vi "ma_Tone estimation (FFT input).vi"(1 "spectral info":T1 {"window" items=["Rectangle"=0, "Hanning"=1, "Hamming"=2, "Blackman-Harris"=3, "Exact Blackman"=4, "Blackman"=5, "Flat Top"=6, "4 Term B-Harris "=7, "7 Term B-Harris"=8, "Low Sidelobe"=9, "Blackman Nuttall"=11, "Triangle"=30, "Bartlett-Hanning"=31, "Bohman"=32, "Parzen"=33, "Welch"=34, "Kaiser"=60, "Dolph-Chebyshev"=61, "Gaussian"=62]}, 2 "three fingers":T3={"f0"=0.0, "df"=1.0, "spectrum"=[]} {"spectrum" format="%.2f"; "df" format="%.2f"; "f0" format="%.2f"}) -> (0 "single tone info.":T2 {"phase [degree]" format="%.2f"; "amplitude" format="%.2f"; "frequency" format="%.5f"})   [LabVIEW 2020, in "NI_MAPro.lvlib"]
doc: "This VI takes the three domainent FFT bins to apply the Newton-Raphson's root finding algorithm to determine the exact frequency, phase and amplitude.\nThe input is not necessary \"three fingers\", it could be two, four, or more."
uses:
  NI_MAPro.lvlib
  ma_sml_Spectrum Cluster (complex).ctl
  ma_sml_Spectral Info.ctl
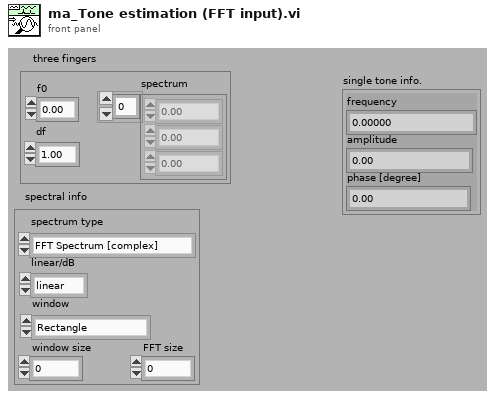
[diagram p1: front panel]
types:
  T1 = typedef "NI_MAPro.lvlib/ma_sml_Spectral Info.ctl" = cluster{"spectrum type":enum16{"FFT Spectrum [complex]", "Amplitude [Magnitude]", "Power [Magnitude^2]", "Cross Spectrum [complex]", "Frequency Response [Complex]"}, "linear/dB":enum16{"linear", "dB"}, "window":u16, "window size":i32, "FFT size":i32}
  T2 = cluster{"frequency":dbl, "amplitude":dbl, "phase [degree]":dbl}
  T3 = typedef "NI_MAPro.lvlib/ma_sml_Spectrum Cluster (complex).ctl" = cluster{"f0":dbl, "df":dbl, "spectrum":cdb[]}
  T4 = cluster{"initial guess frequency":dbl, "Amplitude":dbl, "phase [degree]":dbl}
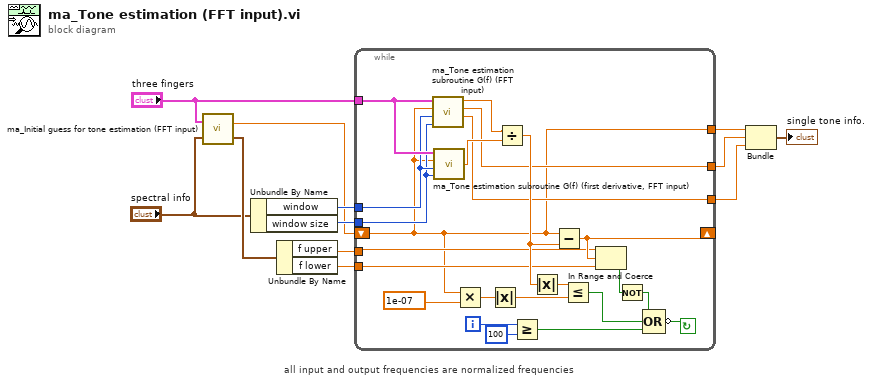
[diagram p0: block diagram]
diagram:
  # "all input and output frequencies are normalized frequencies"
  n1 = call "ma_Initial guess for tone estimation (FFT input).vi"("spectral info"="spectral info", "three fingers"="three fingers") -> ("range"=w6:cluster{"f upper":dbl, "f lower":dbl}, "initial guess frequency"=w1:dbl)
  n2 = Unbundle By Name("spectral info") -> ("window"=w7:u16, "window size"=w8:i32)
  n3 = Unbundle By Name(w6) -> ("f upper"=w5:dbl, "f lower"=w4:dbl)
  n4 = while {
    tunnel: "three fingers" -> [w21]
    tunnel: w4 -> [w22]
    tunnel: w8 -> [w19]
    tunnel: w7 -> [w20]
    tunnel: w5 -> [w23]
    tunnel: [w28] -> w10
    tunnel: [w29] -> w9
    tunnel: [w17] -> w3
    shift-left: w1 -> [w17]
    shift-right: [w25] -> _
    i -> [w18]
    stop <- w31 continue-if-true
    n5 = call "ma_Tone estimation subroutine G(f) (FFT input).vi"("N (window length)"=w19, "window"=w20, "frequency"=w17, "three fingers"=w21) -> ("phase [degree]"=w28:dbl, "Amplitude"=w29:dbl, "G(f)"=w26:dbl)  [unwired: 1 in]
    n6 = call "ma_Tone estimation subroutine G(f) (first derivative, FFT input).vi"("N (window length)"=w19, "window"=w20, "frequency"=w17, "three fingers"=w21) -> ("G'(f)"=w35:dbl)
    n7 = Multiply(x=w17, y=1e-07) -> (x*y=w16:dbl)
    n8 = Absolute Value(x=w16) -> (abs(x)=w13:dbl)
    n9 = Divide(x=w26, y=w35) -> (x/y=w30:dbl)
    n10 = Greater Or Equal?(x=w18, y=100) -> (x >= y?=w32:bool)
    n11 = Absolute Value(x=w30) -> (abs(x)=w33:dbl)
    n12 = Subtract(x=w17, y=w30) -> (x-y=w25:dbl)
    n13 = Less Or Equal?(x=w33, y=w13) -> (x <= y?=w27:bool)
    n14 = In Range and Coerce(upper limit=w23, x=w25, lower limit=w22) -> (In Range?=w24:bool)  [unwired: 1 out]
    n15 = Not(x=w24) -> (.not. x?=w15:bool)
    n16 = Compound Arithmetic op=OR(w15, w27, w32) -> (invert w31:bool)
  }
  n17 = Bundle("initial guess frequency"=w3, "Amplitude"=w9, "phase [degree]"=w10) -> (→"single tone info.":T4)  [unwired: 1 out]
